vi "Select Multiple Objects.vi"   [LabVIEW 2023]
doc: "Demonstrates the use of the Make Selection method in VI Scripting to programmatically select objects on the block diagram."
panel:
  # "Overview: Demonstrates the use of the Make Selection method in VI Scripting to programmatically select objects on the block diagram.\nInstructions:\n1. Open the block diagram of Test - Selection List Target.vi.\n2. Run this VI. All top-level objects on the diagram will become selected. To see this, click the block diagram window title bar of the Test - Selection List Target.vi after running this VI to make it the active window."
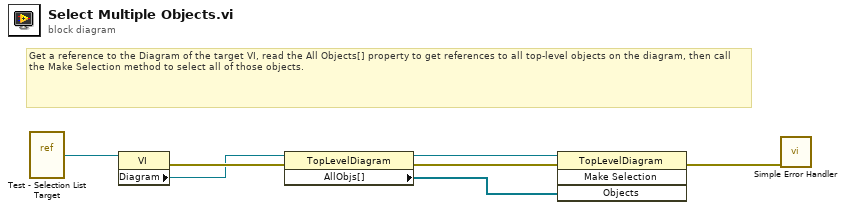
[diagram p0: block diagram]
diagram:
  # "Get a reference to the Diagram of the target VI, read the All Objects[] property to get references to all top-level objects on the diagram, then call the Make Selection method to select all of those objects."
  n1 = vi-ref "Test - Selection List Target.vi"() -> (w7:refnum<vi>)
  n2 = property class="VI"(reference=w7) -> (error out=w6:errorcluster, "Diagram"=w5:refnum<vi>)  [unwired: 1 in, 1 out]
  n3 = property class="TopLevelDiagram"(reference=w5, error in=w6) -> (reference out=w3:refnum<vi>, error out=w4:errorcluster, "AllObjs[]"=w1:refnum<vi>[])
  n4 = invoke class="TopLevelDiagram" method="Make Selection"(reference=w3, error in=w4, "Objects"=w1) -> (error out=w2:errorcluster)  [unwired: 1 in, 3 out]
  n5 = call <vilib>:"Simple Error Handler.vi"("error in (no error)"=w2) -> ()  [unwired: 4 in, 5 out]
